vi "Get FC2 ILC.vi"(11 "Model in":refnum<class "Model.lvclass">) -> (2 "FC2ILC":refnum<class "ILC.lvclass">, 3 "Model out":refnum<class "Model.lvclass">)   [LabVIEW 2015, in "Model.lvclass"]
uses:
  Model.lvclass
  <userlib>/Common/ILC/ILC/ILC.lvclass
  Model.lvclass/Model.ctl
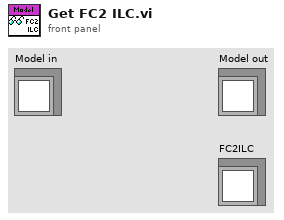
[diagram p1: front panel]
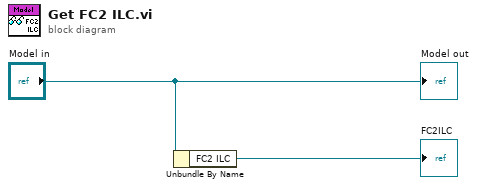
[diagram p0: block diagram]
diagram:
  n1 = Unbundle By Name("Model in") -> ("FC2 ILC"=→"FC2ILC":refnum<class "ILC.lvclass">)
  "Model out" <- "Model in"
